vi "Read XY.vi"(8 "error in (no error)":errorcluster, 11 "VISA resource name":string) -> (0 "error out":errorcluster, 1 "Y mV":dbl, 2 "X mV":dbl, 3 "VISA resource name 2":string, 4 "R":dbl)   [LabVIEW 2024]
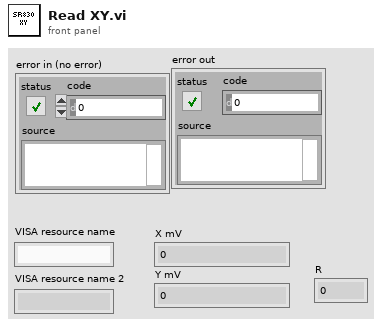
[diagram p1: front panel]
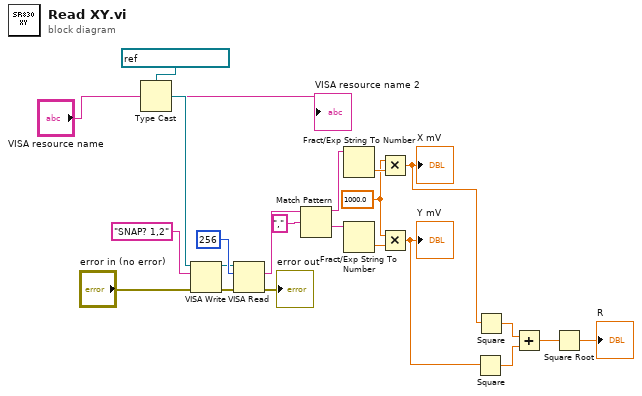
[diagram p0: block diagram]
diagram:
  w10 = 1000.0 ("x")
  n1 = Type Cast(type=refnum<visa-resource-name> "GPIB0::8::INSTR" ("Lockin address 1"), x="VISA resource name") -> (*(type *) &x=w8:refnum<visa-resource-name>)
  n2 = VISA Write(VISA resource name=w8, write buffer="SNAP? 1,2", error in (no error)="error in (no error)") -> (VISA resource name out=w18:refnum<visa-resource-name>, error out=w20:errorcluster)  [unwired: 1 out]
  n3 = VISA Read(VISA resource name=w18, byte count=u32 256, error in (no error)=w20) -> (read buffer=w16:string, error out=→"error out":errorcluster)  [unwired: 2 out]
  n4 = Match Pattern(string=w16, regular expression=",") -> (before substring=w14:string, after substring=w12:string)  [unwired: 1 in, 2 out]
  n5 = Fract/Exp String To Number(string=w14) -> (number=w13:dbl)  [unwired: 3 in, 1 out]
  n6 = Fract/Exp String To Number(string=w12) -> (number=w11:dbl)  [unwired: 3 in, 1 out]
  n7 = Multiply(x=w10, y=w13) -> (x*y=w6:dbl)
  "X mV" <- w6
  n8 = Multiply(x=w10, y=w11) -> (x*y=w5:dbl)
  "Y mV" <- w5
  n9 = Square(x=w5) -> (x^2=w3:dbl)
  n10 = Square(x=w6) -> (x^2=w4:dbl)
  n11 = Add(x=w4, y=w3) -> (x+y=w2:dbl)
  n12 = Square Root(x=w2) -> (sqrt(x)=→"R":dbl)
  "VISA resource name 2" <- "VISA resource name"
